vi "ProdaNG.Process.Get.vi"(8 "error in (no error)":errorcluster, 10 "processId":i32, 11 "dbHandleIn":i32) -> (0 "error out":errorcluster, 1 "Dll Code":i32, 2 "Process":T1, 3 "dbHandle":i32)   [LabVIEW 2016]
doc: "This function returns a product structure for a product, which is identified by a part and a serial number.\nImportant information: The field 'individual' was taken over from the field 'allgemein' of the legacy data directly. Because of this most products have the value 0 further on and only a few the value 1. \nParameter:\nhandle is an Integer, which is returned by the function Login() at the creation of a new connection.\nwabcoPartId is the Id of the part.\nserialNumber is the serial number of the product for the part above.\nproduct is a pointer on a product structure, which is filled if the returncode is 0. The structure must be defined in the calling program.\n\nReturncodes:\n0 No error\n< 0 ORACLE Error code\n6 (ERROR_INVALID_HANDLE) in case of an invalid handle\n1403 Record does not exist"
uses:
  Controls/ProdaNG.Process.ctl
  Controls/ProdaNG.ProcessSize.ctl
  prodllNG.dll
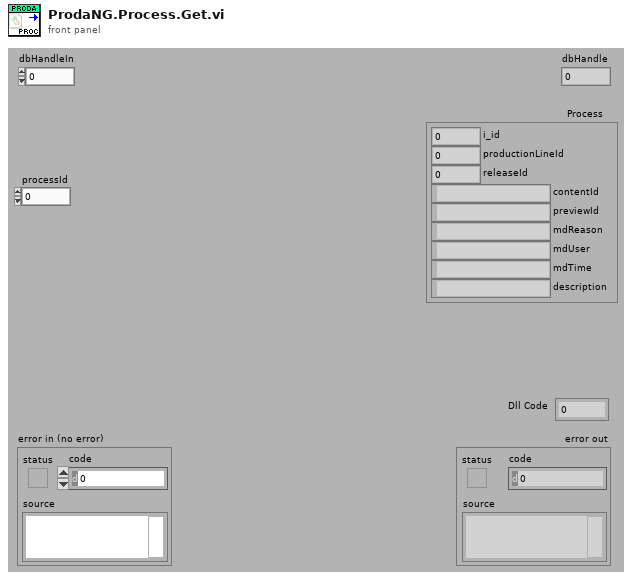
[diagram p1: front panel]
types:
  T1 = typedef "ProdaNG.Process.ctl" = cluster{"i_id":i32, "productionLineId":i32, "releaseId":i32, "contentId":string, "previewId":string, "mdReason":string, "mdUser":string, "mdTime":string, "description":string}
  T2 = typedef "ProdaNG.ProcessSize.ctl" = cluster{"i_id":i32, "productionLineId":i32, "releaseId":i32, "contentId":i32, "previewId":i32, "mdReason":i32, "mdUser":i32, "mdTime":i32, "description":i32}
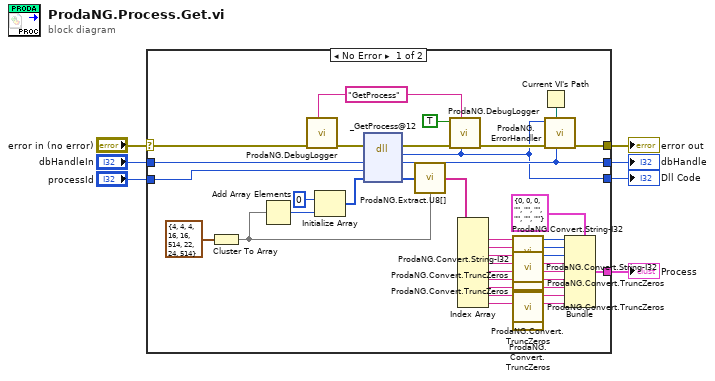
[diagram p0: block diagram]
diagram:
  n1 = case shown="No Error" "error in (no error)" {
    selector: "error in (no error)" -> [w41 w48]
    tunnel: [w46 w48] -> w6
    tunnel: "dbHandleIn" -> [w43 w47]
    tunnel: [w44 w47] -> w4
    tunnel: "processId" -> [w35 _]
    tunnel: [w36 _] -> w2
    tunnel: [w34 _] -> w1
    frame No Error {
      w37 = "GetProcess" ("cmd")
      n2 = Cluster To Array(cluster=T2 {"i_id"=4, "productionLineId"=4, "releaseId"=4, "contentId"=16, "previewId"=16, "mdReason"=514, "mdUser"=22, "mdTime"=24, "description"=514} ("ProcSize")) -> (array=w29:i32[])
      n3 = Add Array Elements(numeric array=w29) -> (sum=w32:i32)
      n4 = call "ProdaNG.DebugLogger.vi"("cmd"=w37, "error in (no error)"=w41) -> ("error out"=w40:errorcluster)  [unwired: 9 in]
      n5 = Initialize Array(u8 0 ("element"), w32) -> (w31:u8[])
      n6 = dll-call lib="D:/svn/LineTraceSystem/SOFTWARE/sources/Database/ProdaNG/prodllNG.dll" fn="_GetProcess@12" ("ProDLL wrapper.dll:ProDLL_wrapper_GetWabcoParts_GetData")(error in=w40, "dbHandle"=w43, "processId"=w35, "process"=w31) -> (error out=w39:errorcluster, "return type"=w36:i32, "dbHandle"=w44:i32, "process"=w30:u8[])  [unwired: 3 in, 1 out]
      n7 = call "ProdaNG.Extract.U8[].vi"("unsigned byte array"=w30, "Sizes"=w29) -> ("Elements"=w13:string[])
      n8 = call "ProdaNG.DebugLogger.vi"("return type"=w36, "cmd"=w37, "error in (no error)"=w39, "done? (F)"=TRUE) -> ("error out"=w38:errorcluster)  [unwired: 7 in]
      n9 = Index Array(array=w13) -> (element #1=w23:string, element #2=w22:string, element #3=w27:string, element #4=w12:string, element #5=w11:string, element #6=w10:string, element #7=w9:string, element #8=w21:string, element #9=w19:string)  [unwired: 9 in]
      n10 = call "ProdaNG.Convert.String-I32.vi"("unsigned byte string"=w23) -> ("32bit integer"=w25:i32)  [unwired: 10 in]
      n11 = call "ProdaNG.Convert.String-I32.vi"("unsigned byte string"=w22) -> ("32bit integer"=w24:i32)  [unwired: 10 in]
      n12 = call "ProdaNG.Convert.String-I32.vi"("unsigned byte string"=w27) -> ("32bit integer"=w26:i32)  [unwired: 10 in]
      n13 = call "ProdaNG.Convert.TruncZeros.vi"("string with \\0s"=w12) -> ("LV string"=w17:string)  [unwired: 10 in]
      n14 = call "ProdaNG.Convert.TruncZeros.vi"("string with \\0s"=w11) -> ("LV string"=w16:string)  [unwired: 10 in]
      n15 = call "ProdaNG.Convert.TruncZeros.vi"("string with \\0s"=w10) -> ("LV string"=w14:string)  [unwired: 10 in]
      n16 = call "ProdaNG.Convert.TruncZeros.vi"("string with \\0s"=w9) -> ("LV string"=w15:string)  [unwired: 10 in]
      n17 = call "ProdaNG.Convert.TruncZeros.vi"("string with \\0s"=w21) -> ("LV string"=w20:string)  [unwired: 10 in]
      n18 = call "ProdaNG.Convert.TruncZeros.vi"("string with \\0s"=w19) -> ("LV string"=w18:string)  [unwired: 10 in]
      n19 = Current VI's Path() -> (path=w45:path)
      n20 = call "ProdaNG.ErrorHandler.vi"("dbHandleIn"=w44, "Path"=w45, "error in"=w38, "output_parameter"=w36) -> ("error out"=w46:errorcluster)  [unwired: 7 in]
      n21 = Bundle(cluster=T1 {"i_id"=0, "productionLineId"=0, "releaseId"=0, "contentId"="", "previewId"="", "mdReason"="", "mdUser"="", "mdTime"="", "description"=""} ("ProcessStep"), "i_id"=w25, "productionLineId"=w24, "releaseId"=w26, "contentId"=w17, "previewId"=w16, "mdReason"=w14, "mdUser"=w15, "mdTime"=w20, "description"=w18) -> (w34:T1)
    }
    frame Error {
    }
  }
  "error out" <- w6
  "dbHandle" <- w4
  "Dll Code" <- w2
  "Process" <- w1
